vi "GyroActions.vi"(6 "Zero":bool, 7 "Update":bool, 10 "YRPHfH_in":T3, 11 "navX Device":T1={"Interface"={"Protocol"=enum."SERIAL", "Update Rate (4Hz-60Hz)"=4, "navX Open TypeDef"=variant}, "Notify Packet"=refnum, "Loop VI Refnum"=refnum, "Ready to Close Occurrence Refnum"=refnum} {"Interface"."Update Rate (4Hz-60Hz)" min=4 max=60 step=1}) -> (0 "Pitch":dbl, 1 "Yaw":dbl, 2 "YRPHfH_out":T3, 3 "navX Device":T1={"Interface"={"Protocol"=enum."SERIAL", "Update Rate (4Hz-60Hz)"=4, "navX Open TypeDef"=variant}, "Notify Packet"=refnum, "Loop VI Refnum"=refnum, "Ready to Close Occurrence Refnum"=refnum} {"Interface"."Update Rate (4Hz-60Hz)" min=4 max=60 step=1}, 4 "Roll":dbl)   [LabVIEW 2015]
uses:
  navX Library v2/TypeDefs/Z900_navX_DeviceTypeDef.ctl
  navX Library v2/TypeDefs/Z900_navX_ProtocolTypeDef.ctl
  navX Library v2/TypeDefs/Z900_navX_NotifyPacketTypeDef.ctl
  navX Library v2/TypeDefs/Z900_navX_ActionTypeDef.ctl
  navX Library v2/navX Library v2.lvlib
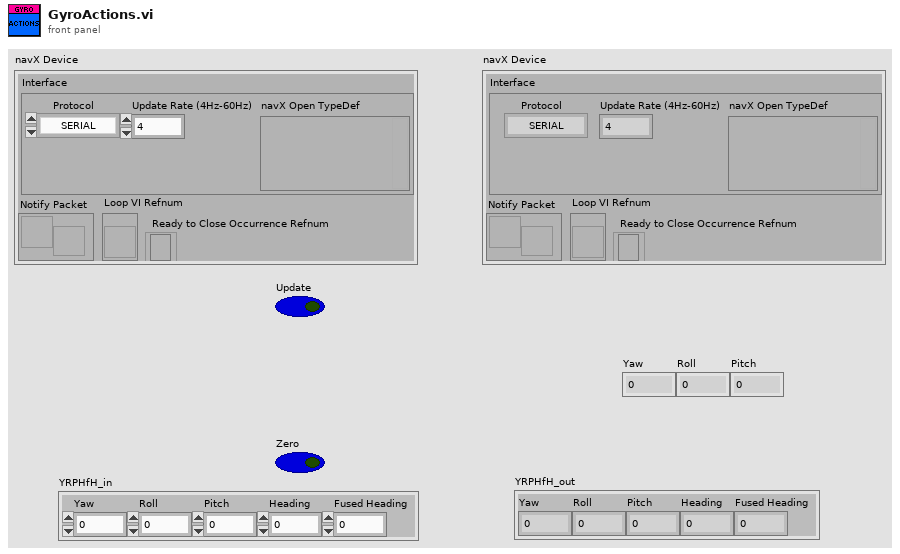
[diagram p1: front panel]
types:
  T1 = typedef "navX Library v2.lvlib/Z900_navX_DeviceTypeDef.ctl" = cluster{"Interface":cluster{"Protocol":T2, "Update Rate (4Hz-60Hz)":u8, "navX Open TypeDef":variant}, "Notify Packet":refnum<notifier>, "Loop VI Refnum":refnum<vi>, "Ready to Close Occurrence Refnum":refnum<k4>}
  T2 = typedef "navX Library v2.lvlib/Z900_navX_ProtocolTypeDef.ctl" = enum16{"SERIAL", "I2C", "SPI"}
  T3 = cluster{"Yaw":dbl, "Roll":dbl, "Pitch":dbl, "Heading":dbl, "Fused Heading":dbl}
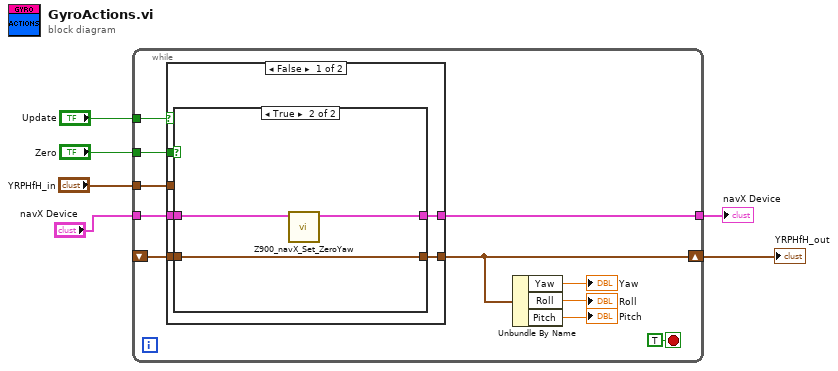
[diagram p0: block diagram]
diagram:
  n1 = while {
    tunnel: "YRPHfH_in" -> [w13]
    shift-right: [w12] -> w3
    shift-left: _ -> [w15]
    tunnel: "Update" -> [w16]
    tunnel: "Zero" -> [w14]
    tunnel: "navX Device" -> [w11]
    tunnel: [w10] -> w1
    stop <- TRUE stop-if-true
    n2 = case shown="False" w16 {
      tunnel: w15 -> [w21 _]
      tunnel: w14 -> [w22 _]
      tunnel: [w20 w29] -> w12
      tunnel: w13 -> [_ w29]
      tunnel: w11 -> [w19 w28]
      tunnel: [w18 w28] -> w10
      frame False {
        n3 = case shown="True" w22 {
          tunnel: w21 -> [w24 w27]
          tunnel: [w24 w27] -> w20
          tunnel: w19 -> [w23 w26]
          tunnel: [w23 w25] -> w18
          frame False {
          }
          frame True {
            n4 = call "Z900_navX_Set_ZeroYaw.vi"("navX Device"=w26) -> ("navX Device"=w25:T1)  [unwired: 9 in, 1 out]
          }
        }
      }
      frame True {
      }
    }
    n5 = Unbundle By Name(w12) -> ("Yaw"=→"Yaw":dbl, "Roll"=→"Roll":dbl, "Pitch"=→"Pitch":dbl)
  }
  "YRPHfH_out" <- w3
  "navX Device" <- w1
